vi "Set_Tree_Item_Proj_Folder.vi"(8 "error in (no error)":errorcluster, 11 "IB_TreeProjFolderItem in":refnum<class "IB_Tree_Item_Proj_Folder.lvclass">) -> (0 "error out":errorcluster, 3 "IB_TreeProjFolderItem out":refnum<class "IB_Tree_Item_Proj_Folder.lvclass">)   [LabVIEW 2020, in "IB_Tree_Item_Proj_Folder.lvclass"]
uses:
  <vilib>/AppBuilder/IB_Classes/Tree_Item_Proj_Folder/IB_Tree_Item_Proj_Folder.lvclass
  <vilib>/AppBuilder/IB_Classes/Tree_Item_Proj_Folder/IB_Tree_Item_Proj_Folder.lvclass/IB_Tree_Item_Proj_Folder.ctl
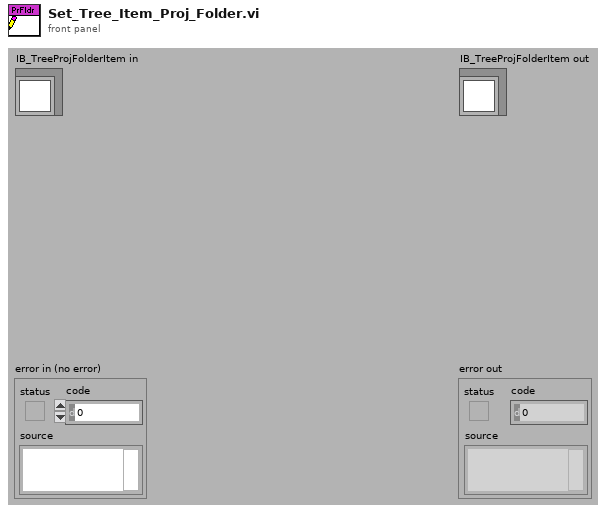
[diagram p1: front panel]
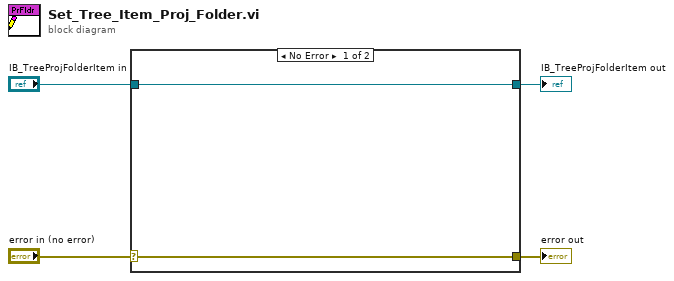
[diagram p0: block diagram]
diagram:
  n1 = case shown="No Error" "error in (no error)" {
    selector: "error in (no error)" -> [w6 w7]
    tunnel: [w6 w7] -> w3
    tunnel: [w5 w8] -> w1
    tunnel: "IB_TreeProjFolderItem in" -> [w5 w8]
    frame No Error {
    }
    frame Error {
    }
  }
  "error out" <- w3
  "IB_TreeProjFolderItem out" <- w1
